vi "半周期测量_连续.vi"() -> ()   [LabVIEW 2013]
uses:
  <userlib>/ArtDAQ/_SubVI/ArtDAQ_CreateCISemiPeriodChan.vi
  <userlib>/ArtDAQ/_SubVI/ArtDAQ_CfgImplicitTiming.vi
  <userlib>/ArtDAQ/_SubVI/ArtDAQ_Read Counter DBL NSamp.vi
panel:
  in  "每通道点数":i32=100
  in  "Stop":bool
  out "数据":dbl[](array[numeric])
  in  "计数器":string="Dev1/ctr0"
  in  "最小测量值":dbl=1e-06 format="%0.6f"
  in  "最大测量值":dbl=10.0 format="%0.6f"
  out "错误输出":errorcluster
  # "通道属性"
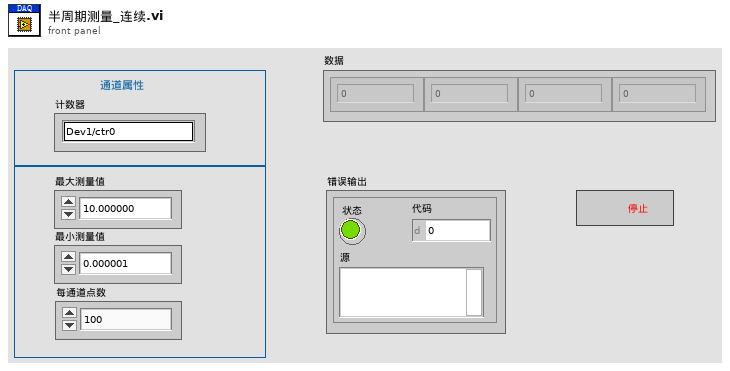
[diagram p1: front panel]
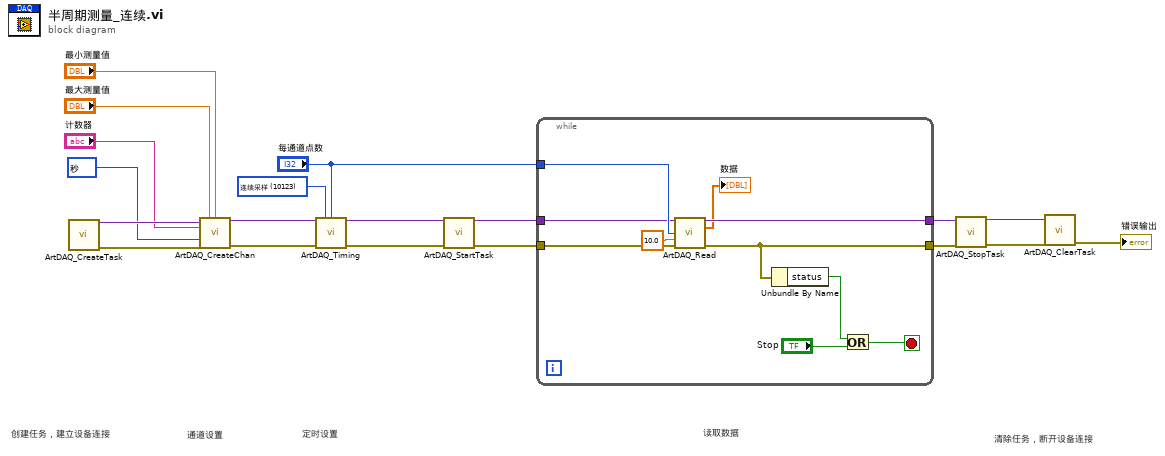
[diagram p0: block diagram]
diagram:
  w6 = 10123 items=["有限点采样"=10178, "连续采样"=10123] ("SampleMode")
  w9 = 10364 items=["秒"=10364, "时钟滴答"=10304, "来自自定义换算"=10065] ("Units")
  # "清除任务，断开设备连接"
  # "读取数据"
  # "定时设置"
  # "通道设置"
  # "创建任务，建立设备连接"
  n1 = call <userlib>:"ArtDAQ_CreateTask.vi"() -> ("任务句柄"=w19:variant, "错误输出"=w18:errorcluster)  [unwired: 14 in]
  n2 = call-poly <userlib>:"ArtDAQ_CreateChan.vi"("任务句柄"=w19, "最大值"="最大测量值", "最小值"="最小测量值", "计数器"="计数器", "单位"=w9, "错误输入"=w18) -> ("任务句柄"=w8:variant, "错误输出"=w7:errorcluster)  [unwired: 8 in]
  n3 = call-poly <userlib>:"ArtDAQ_Timing.vi"("任务句柄"=w8, "采样模式"=w6, "每通道采样数"="每通道点数", "错误输入"=w7) -> ("任务句柄"=w4:variant, "错误输出"=w3:errorcluster)  [unwired: 10 in]
  n4 = call <userlib>:"ArtDAQ_StartTask.vi"("任务句柄"=w4, "错误输入"=w3) -> ("任务句柄"=w2:variant, "错误输出"=w1:errorcluster)  [unwired: 12 in]
  n5 = while {
    tunnel: [w29] -> w16
    tunnel: [w28] -> w14
    tunnel: "每通道点数" -> [w27]
    tunnel: w2 -> [w22]
    tunnel: w1 -> [w21]
    stop <- w20 stop-if-true
    n6 = call-poly <userlib>:"ArtDAQ_Read.vi"("任务句柄"=w22, "每通道采样数"=w27, "超时s"=10.0 ("Timeout"), "错误输入"=w21) -> ("任务句柄"=w29:variant, "数据"=→"数据":dbl[], "错误输出"=w28:errorcluster)  [unwired: 8 in, 1 out]
    n7 = Unbundle By Name(w28) -> ("status"=w24:bool)
    n8 = Or(x=w24, y="Stop") -> (x .or. y?=w20:bool)
  }
  n9 = call <userlib>:"ArtDAQ_StopTask.vi"("任务句柄"=w16, "错误输入"=w14) -> ("任务句柄"=w15:variant, "错误输出"=w13:errorcluster)  [unwired: 12 in]
  n10 = call <userlib>:"ArtDAQ_ClearTask.vi"("任务句柄"=w15, "错误输入"=w13) -> ("错误输出"=→"错误输出":errorcluster)  [unwired: 13 in]
